vi "DMMs_initialize.vi"(6 "RunIdentifier":string, 7 "InstName":string, 8 "error in (no error)":errorcluster, 9 "base path":path, 10 "DMMsConfig":T1(array[cluster]), 11 "DMMsData in":refnum<class "DMMsData.lvclass">) -> (0 "error out":errorcluster, 1 "DMMsLabels":string[](array[string]), 3 "DMMsData out":refnum<class "DMMsData.lvclass">)   [LabVIEW 2017, in "DMMsData.lvclass"]
uses:
  DMMsData.lvclass
  DMMsData.lvclass/DMMsData.ctl
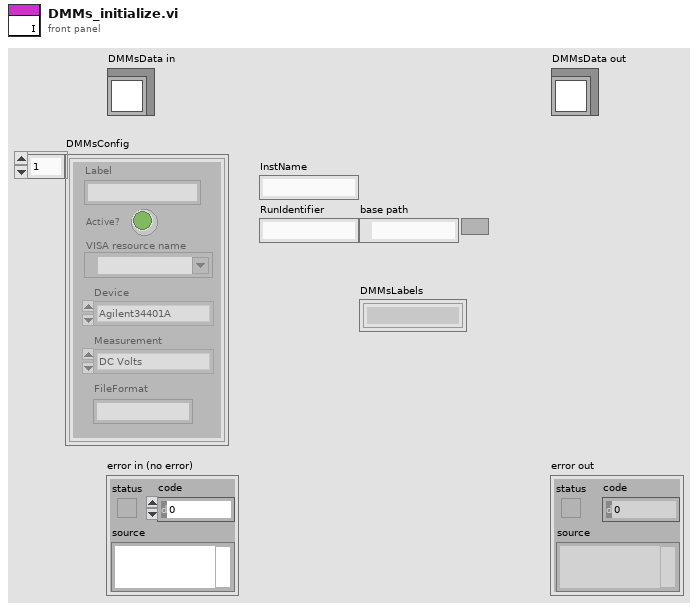
[diagram p1: front panel]
types:
  T1 = cluster{"Label":string, "Active?":bool, "VISA resource name":refnum<visa-resource-name>, "Device":enum16{"Agilent34401A", "ADCMT7351", "HP3478A"}, "Measurement":enum16{"DC Volts", "DC Currents", "2-Wire Resistance", "4-Wire Resistance"}, "FileFormat":string}[]
  T2 = enum16{"open", "replace", "create", "open or create", "replace or create", "replace or create with confirmation"}
  T3 = enum16{"DC Volts", "DC Currents", "2-Wire Resistance", "4-Wire Resistance"}
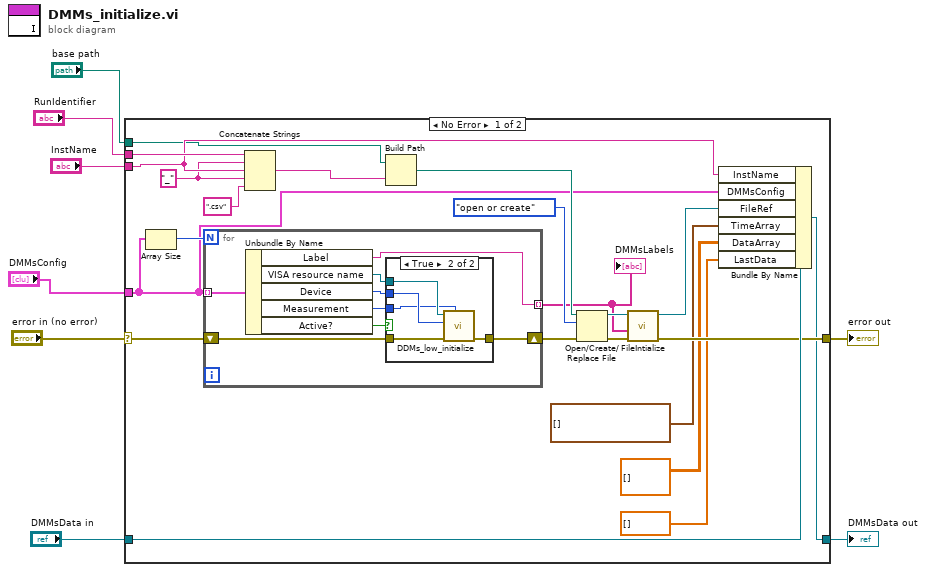
[diagram p0: block diagram]
diagram:
  n1 = case shown="No Error" "error in (no error)" {
    selector: "error in (no error)" -> [w21 w46]
    tunnel: [w18 w46] -> w7
    tunnel: [w9 w45] -> w5
    tunnel: "DMMsData in" -> [w30 w45]
    tunnel: "DMMsConfig" -> [w13 _]
    tunnel: "InstName" -> [w27 _]
    tunnel: "RunIdentifier" -> [w28 _]
    tunnel: "base path" -> [w26 _]
    frame No Error {
      w11 = "_" ("string")
      n2 = Array Size(array=w13) -> (size(s)=w29:i32)
      n3 = for {
        N: w29 -> [_]
        tunnel: [w38] -> w12 mode=indexing
        shift-right: [w33] -> w20
        shift-left: w21 -> [w34]
        tunnel: w13 -> [w32] mode=indexing
        n4 = Unbundle By Name(w32) -> ("Label"=w38:string, "VISA resource name"=w37:refnum<visa-resource-name>, "Device"=w36:enum16{"Agilent34401A", "ADCMT7351", "HP3478A"}, "Measurement"=w35:T3, "Active?"=w31:bool)
        n5 = case shown="True" w31 {
          tunnel: w37 -> [_ w42]
          tunnel: w36 -> [_ w41]
          tunnel: w35 -> [_ w40]
          tunnel: w34 -> [w39 w44]
          tunnel: [w39 w43] -> w33
          frame False {
          }
          frame True {
            n6 = call "DDMs_low_initialize.vi"("Measurement"=w40, "error in (no error)"=w44, "Device"=w41, "VISA resource name"=w42) -> ("error out"=w43:errorcluster)  [unwired: 6 in, 1 out]
          }
        }
      }
      "DMMsLabels" <- w12
      n7 = Concatenate Strings(w28, w11, w27, w11, ".csv" ("string")) -> (w25:string)
      n8 = Build Path(base path=w26, name or relative path=w25) -> (appended path=w24:path)
      n9 = Open/Create/Replace File(file path (use dialog)=w24, error in=w20, operation (0:open)=T2."open or create") -> (refnum out=w22:refnum<file>, error out=w19:errorcluster)  [unwired: 3 in, 1 out]
      n10 = call "FileIntialize.vi"("Error In"=w19, "Labels"=w12, "refnum in"=w22) -> ("Error Out"=w18:errorcluster, "File Refnum"=w17:refnum<file>)  [unwired: 7 in]
      n11 = Bundle By Name(cluster=w30, "InstName"=w27, "DMMsConfig"=w13, "FileRef"=w17, "TimeArray"=timestamp[] [], "DataArray"=dbl[][] [], "LastData"=dbl[] []) -> (w9:refnum<class "DMMsData.lvclass">)
    }
    frame Error {
    }
  }
  "error out" <- w7
  "DMMsData out" <- w5
